vi "web.vi"(8 "error in":errorcluster caption="错误输入", 9 "Password":string="88888888", 10 "Delay":u32=3000, 11 "WIFIName":string="Honor V10") -> (0 "错误输出":errorcluster, 1 "time":u64, 2 "TotalOut":string, 3 "PASS？":bool)   [LabVIEW 2013]
panel:
  in  "FAIL":bool
  in  "PASS":bool
  out "outerText":string
  out "outerHTML":string
  in  "WebBrowser":refnum<k7>(container)
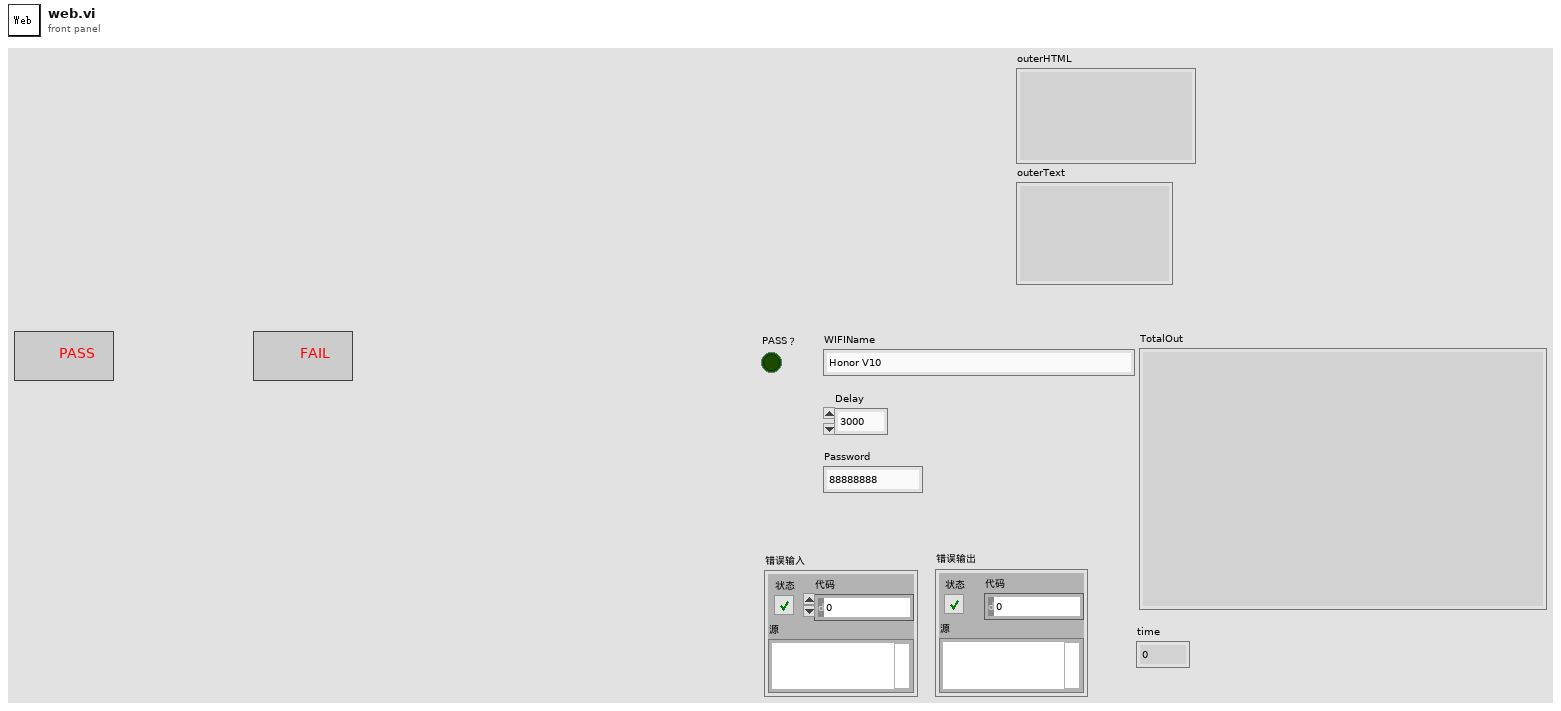
[diagram p1: front panel]
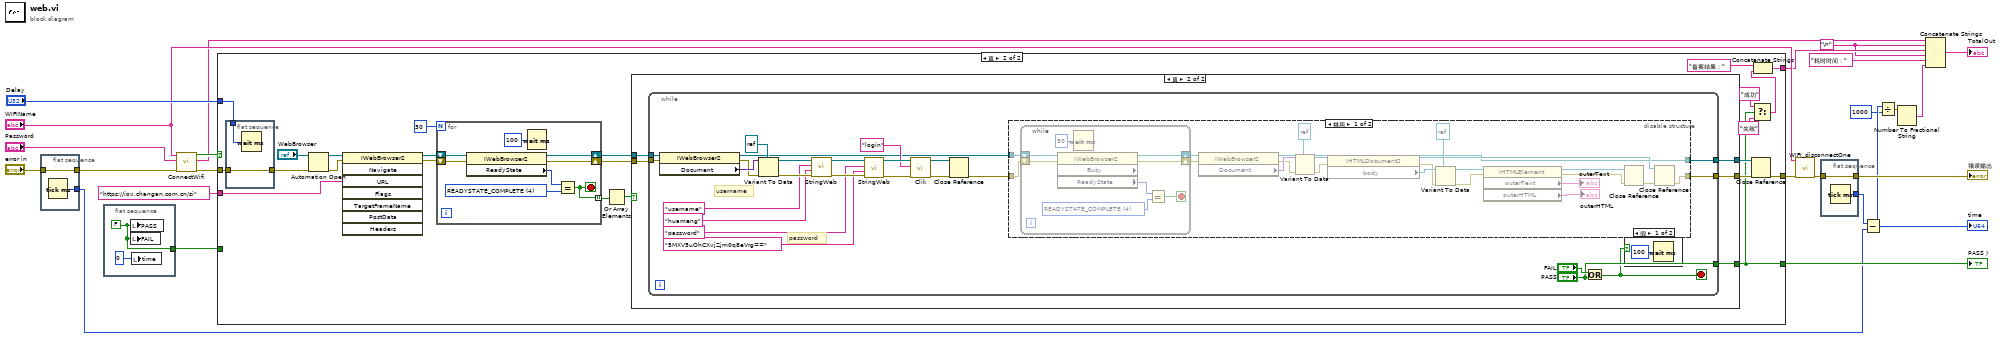
[diagram p0: block diagram]
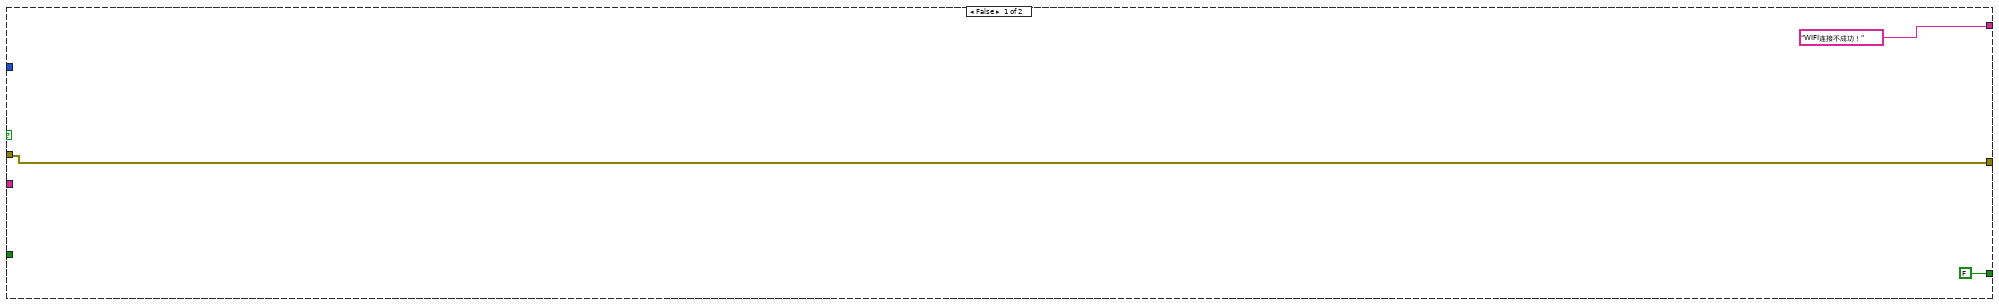
[diagram p2: hidden frame]
diagram:
  w6 = "\n"
  n1 = flat-sequence {
    tunnel: [w26] -> w15
    tunnel: "error in" -> [w26]
    tunnel: [w25] -> w10
    frame #0 {
      n2 = Tick Count (ms)() -> (millisecond timer value=w25:u32)
    }
  }
  n3 = flat-sequence {
    tunnel: [w28] -> w16
    frame #0 {
      w28 = FALSE
      n4 = local write "PASS"(w28) -> ()
      n5 = local write "FAIL"(w28) -> ()
      n6 = local write "time"(0) -> ()
    }
  }
  n7 = call "ConnectWifi.vi"("error in"=w15, "Password"="Password", "WIFIName"="WIFIName") -> ("error out"=w21:errorcluster, "TotalOut"=w9:string, "Acess"=w22:bool)  [unwired: 5 in, 1 out]
  n8 = case shown="真" w22 {
    tunnel: [w31 w46] -> w18
    tunnel: [FALSE w36] -> w24
    tunnel: w21 -> [w31 w39]
    tunnel: "https://iov.changan.com.cn/si" ("URL") -> [_ w41]
    tunnel: "Delay" -> [_ w38]
    tunnel: w16 -> [_ _]
    tunnel: ["WIFI连接不成功！" w32] -> w8
    frame False {
    }
    frame True {
      n9 = flat-sequence {
        tunnel: [w56] -> w40
        tunnel: w39 -> [w56]
        tunnel: w38 -> [w55]
        frame #0 {
          n10 = Wait (ms)(milliseconds to wait=w55) -> ()  [unwired: 1 out]
        }
      }
      n11 = Automation Open(error in (no error)=w40, Automation Refnum="WebBrowser") -> (Automation Refnum=w53:refnum<k7>, error out=w42:errorcluster)  [unwired: 2 in]
      n12 = invoke on="调用节点" class="IWebBrowser2" method="Navigate"(reference=w53, error in=w42, "URL"=w41) -> (reference out=w52:refnum<k7>, error out=w51:errorcluster)  [unwired: 5 in, 6 out]
      n13 = for {
        N: 30 -> [_]
        shift-right: [w124] -> w50
        shift-left: w52 -> [w129]
        shift-right: [w123] -> w49
        shift-left: w51 -> [w128]
        tunnel: [w122] -> w44 mode=indexing
        stop <- w122 stop-if-true
        w125 = 4 items=["READYSTATE_UNINITIALIZED", "READYSTATE_LOADING", "READYSTATE_LOADED", "READYSTATE_INTERACTIVE", "READYSTATE_COMPLETE"] ("ReadyState")
        n14 = property on="属性节点" class="IWebBrowser2"(reference=w129, error in=w128) -> (reference out=w124:refnum<k7>, error out=w123:errorcluster, "ReadyState"=w126:i32)
        n15 = Wait (ms)(milliseconds to wait=u32 100 ("等待时间（毫秒）")) -> ()  [unwired: 1 out]
        n16 = Equal?(x=w126, y=w125) -> (x = y?=w122:bool)
      }
      n17 = Or Array Elements(Boolean array=w44) -> (logical OR=w43:bool)
      n18 = case shown="真" w43 {
        tunnel: w50 -> [w58 w63]
        tunnel: w49 -> [w57 w62]
        tunnel: [w57 w61] -> w48
        tunnel: [w58 w60] -> w47
        tunnel: [_ w59] -> w36
        frame False {
        }
        frame True {
          n19 = while {
            tunnel: w63 -> [w88]
            tunnel: w62 -> [w87]
            tunnel: [w68] -> w61
            tunnel: [w67] -> w60
            tunnel: ["PASS"] -> w59
            stop <- w64 stop-if-true
            # "password"
            # "username"
            n20 = property on="属性节点" class="IWebBrowser2"(reference=w88, error in=w87) -> (reference out=w70:refnum<k7>, error out=w84:errorcluster, "Document"=w86:variant)
            n21 = Variant To Data(error in=w84, type=refnum<k7> refnum ("类型"), Variant=w86) -> (data=w83:refnum<k7>, error out=w85:errorcluster)
            n22 = call "StringWeb.vi"("错误输入"=w85, "value"="huameng", "string in"="username", "refnum in"=w83) -> ("错误输出"=w79:errorcluster, "refnum out"=w78:refnum<k7>)  [unwired: 6 in]
            n23 = call "StringWeb.vi"("错误输入"=w79, "value"="5MXV5uOhCXvjZjm0q8eVrg==", "string in"="password", "refnum in"=w78) -> ("错误输出"=w75:errorcluster, "refnum out"=w74:refnum<k7>)  [unwired: 6 in]
            n24 = call "Clik.vi"("refnum in"=w74, "string in"="login", "错误输入"=w75) -> ("refnum out"=w71:refnum<k7>, "错误输出"=w72:errorcluster)  [unwired: 6 in]
            n25 = Close Reference(reference=w71, error in (no error)=w72) -> (error out=w69:errorcluster)
            n26 = disable-structure shown="禁用" {
              disable-tunnel: w70 -> [w111 w120]
              disable-tunnel: w69 -> [w110 w121]
              disable-tunnel: [w91 w121] -> w68
              disable-tunnel: [w90 w120] -> w67
              frame Disabled {
                n27 = while {
                  shift-right: [w113] -> w109
                  shift-left: w111 -> [w119]
                  shift-right: [w114] -> w108
                  shift-left: w110 -> [w118]
                  stop <- w115 stop-if-true
                  w116 = 4 items=["READYSTATE_UNINITIALIZED", "READYSTATE_LOADING", "READYSTATE_LOADED", "READYSTATE_INTERACTIVE", "READYSTATE_COMPLETE"] ("ReadyState")
                  n28 = property on="属性节点" class="IWebBrowser2" props=["Busy", "ReadyState"](reference=w119, error in=w118) -> (reference out=w113:refnum<k7>, error out=w114:errorcluster, "ReadyState"=w117:i32)  [unwired: 1 out]
                  n29 = Wait (ms)(milliseconds to wait=u32 50 ("等待时间（毫秒）")) -> ()  [unwired: 1 out]
                  n30 = Equal?(x=w117, y=w116) -> (x = y?=w115:bool)
                }
                n31 = property on="属性节点" class="IWebBrowser2"(reference=w109, error in=w108) -> (reference out=w90:refnum<k7>, error out=w106:errorcluster, "Document"=w107:variant)
                n32 = Variant To Data(error in=w106, type=refnum<k7> refnum ("引用输出"), Variant=w107) -> (data=w104:refnum<k7>, error out=w103:errorcluster)
                n33 = property on="属性节点" class="IHTMLDocument2"(reference=w104, error in=w103) -> (reference out=w92:refnum<k7>, error out=w98:errorcluster, "body"=w99:refnum<k7>)
                n34 = Variant To Data(error in=w98, type=refnum<k7> refnum ("引用输出"), Variant=w99) -> (data=w101:refnum<k7>, error out=w100:errorcluster)
                n35 = property on="属性节点" class="IHTMLElement"(reference=w101, error in=w100) -> (reference out=w95:refnum<k7>, error out=w94:errorcluster, "outerText"=→"outerText":string, "outerHTML"=→"outerHTML":string)
                n36 = Close Reference(reference=w95, error in (no error)=w94) -> (error out=w93:errorcluster)
                n37 = Close Reference(reference=w92, error in (no error)=w93) -> (error out=w91:errorcluster)
              }
              frame Enabled {
              }
            }
            n38 = Or(x="FAIL", y="PASS") -> (x .or. y?=w64:bool)
            n39 = case shown="假" w64 {
              frame False {
                n40 = Wait (ms)(milliseconds to wait=u32 100 ("等待时间（毫秒）")) -> ()  [unwired: 1 out]
              }
              frame True {
              }
            }
          }
        }
      }
      n41 = Close Reference(reference=w47, error in (no error)=w48) -> (error out=w46:errorcluster)
      n42 = Select(t="成功", s=w36, f="失败") -> (s? t:f=w33:string)
      n43 = Concatenate Strings("备案结果：", w33) -> (w32:string)
    }
  }
  "PASS？" <- w24
  n44 = call "WIFI_disconnectOne.vi"("错误输入"=w18, "WIFI_Name"="WIFIName") -> ("error out"=w13:errorcluster)  [unwired: 8 in, 1 out]
  n45 = flat-sequence {
    tunnel: [w131] -> w12
    tunnel: w13 -> [w131]
    tunnel: [w130] -> w11
    frame #0 {
      n46 = Tick Count (ms)() -> (millisecond timer value=w130:u32)
    }
  }
  n47 = Subtract(x=w11, y=w10) -> (x-y=w5:u32)
  "time" <- w5
  n48 = Divide(x=w5, y=u32 1000) -> (x/y=w3:dbl)
  n49 = Number To Fractional String(number=w3) -> (F-format string=w1:string)  [unwired: 3 in]
  n50 = Concatenate Strings(w9, w6, w8, w6, "耗时时间：", w1) -> (→"TotalOut":string)
  "错误输出" <- w12
